vi "HDEL.vi"(8 "error in (no error)":errorcluster, 9 "fields":string[](array[string]), 10 "key":string, 11 "Redis Client in":refnum<class "Redis Client.lvclass">) -> (0 "error out":errorcluster, 2 "# removed":i64, 3 "Redis Client out":refnum<class "Redis Client.lvclass">)   [LabVIEW 2019, in "Redis Client for LabVIEW.lvlib" / "Redis Client.lvclass"]
uses:
  Redis Client.lvclass
  lib/RESP3-for-LabVIEW/RESP3/high-level/RESP3 Make Bulk String.vi
  lib/RESP3-for-LabVIEW/RESP3/subVIs/RESP3 Make String Base.vi
  lib/RESP3-for-LabVIEW/RESP3/types/RESP3 data type attribute.vi
  lib/RESP3-for-LabVIEW/RESP3/high-level/RESP3 Make Array.vi
  lib/RESP3-for-LabVIEW/RESP3/high-level/RESP3 Get Integer.vi
  lib/RESP3-for-LabVIEW/RESP3/RESP3.lvlib
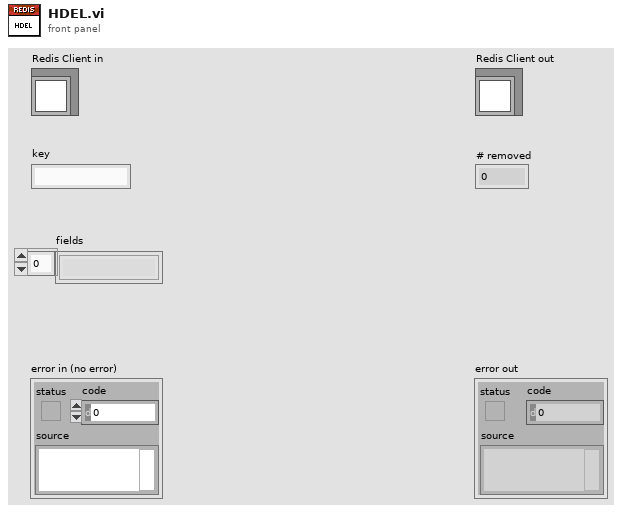
[diagram p1: front panel]
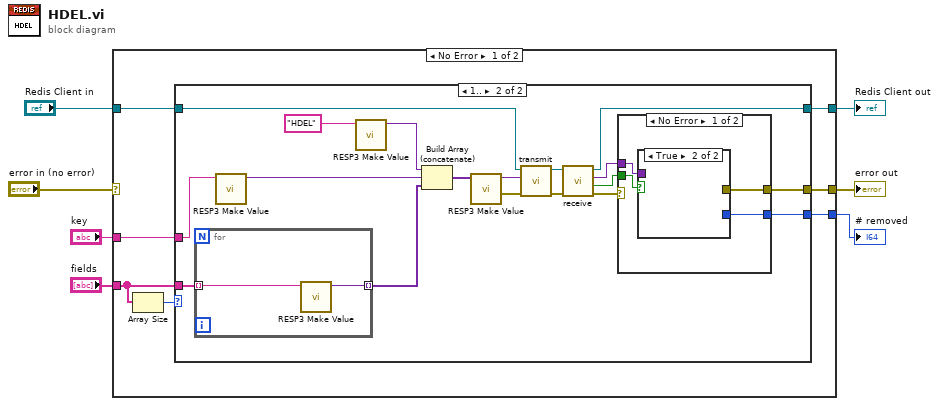
[diagram p0: block diagram]
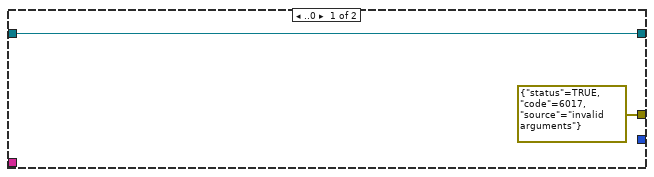
[diagram p2: hidden frame]
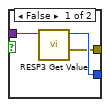
[diagram p3: hidden frame]
diagram:
  n1 = case shown="No Error" "error in (no error)" {
    selector: "error in (no error)" -> [_ w46]
    tunnel: [w10 w46] -> w6
    tunnel: "Redis Client in" -> [w14 w45]
    tunnel: [w12 w45] -> w4
    tunnel: "key" -> [w13 _]
    tunnel: "fields" -> [w9 _]
    tunnel: [w11 _] -> w1
    frame No Error {
      n2 = Array Size(array=w9) -> (size(s)=w8:i32)
      n3 = case shown="1.." w8 {
        tunnel: w14 -> [w16 w34]
        tunnel: w13 -> [_ w23]
        tunnel: [w16 w30] -> w12
        tunnel: [_ w24] -> w11
        tunnel: [errorcluster {"status"=TRUE, "code"=6017, "source"="invalid arguments"} ("error IO") w25] -> w10
        tunnel: w9 -> [_ w29]
        frame ..0 {
        }
        frame 1.. {
          n4 = for {
            tunnel: w29 -> [w44] mode=indexing
            tunnel: [w43] -> w33 mode=indexing
            n5 = call-poly "RESP3 Make Value.vi"("String"=w44) -> ("RESP3 Value out"=w43:variant)  [unwired: 9 in, 1 out]
          }
          n6 = call-poly "RESP3 Make Value.vi"("String"=w23) -> ("RESP3 Value out"=w20:variant)  [unwired: 9 in, 1 out]
          n7 = call-poly "RESP3 Make Value.vi"("String"="HDEL" ("string in")) -> ("RESP3 Value out"=w21:variant)  [unwired: 9 in, 1 out]
          n8 = Build Array (concatenate)(w21, w20, w33) -> (w19:variant[])
          n9 = call-poly "RESP3 Make Value.vi"("RESP3 Values in"=w19) -> ("error out"=w18:errorcluster, "RESP3 Value out"=w17:variant)  [unwired: 9 in]
          n10 = call-dynamic "transmit.vi"("error in (no error)"=w18, "RESP3 Value"=w17, "Redis Client in"=w34) -> ("error out"=w31:errorcluster, "Redis Client out"=w32:refnum<class "Redis Client.lvclass">)  [unwired: 7 in]
          n11 = call-dynamic "receive.vi"("error in (no error)"=w31, "Redis Client in"=w32) -> ("error out"=w26:errorcluster, "timed out?"=w27:bool, "RESP3 Value"=w28:variant, "Redis Client out"=w30:refnum<class "Redis Client.lvclass">)  [unwired: 6 in]
          n12 = case shown="No Error" w26 {
            selector: w26 -> [_ w42]
            tunnel: [w38 _] -> w24
            tunnel: [w37 w42] -> w25
            tunnel: w28 -> [w36 _]
            tunnel: w27 -> [w35 _]
            frame No Error {
              n13 = case shown="True" w35 {
                tunnel: [w40 _] -> w38
                tunnel: [w39 _] -> w37
                tunnel: w36 -> [w41 _]
                frame False {
                  n14 = call-poly "RESP3 Get Value.vi"("RESP3 Value in"=w41) -> ("error out"=w39:errorcluster, "I64 out"=w40:i64)  [unwired: 8 in, 1 out]
                }
                frame True {
                }
              }
            }
            frame Error {
            }
          }
        }
      }
    }
    frame Error {
    }
  }
  "error out" <- w6
  "Redis Client out" <- w4
  "# removed" <- w1
